vi "Zaber Beginner - Send Commands in a Loop.vi"() -> ()   [LabVIEW 2020]
doc: "You can repeat commands using for loop or while loop structures. This example shows how to use a for loop to replace the five <code>Move Relative -10000</code> commands in the previous example.\nNote that the error line needs to use a shift register in the loop, so that an error will get carried forward through later iterations.\nNow that you've seen two, here are some features common to most of our examples:\n* Place error and COM port wires in a straight line across the bottom. This is the main data flow of the diagram.\n* Start with Initialize to set timeouts and other things, and end with Close. If you don't use Close, Labview won't complain but other applications won't be able to use the COM port."
uses:
  Public/Utility/Request.ctl
  ZaberTSeries.lvlib
panel:
  in  "VISA resource name":refnum<visa-resource-name>
  # "This behaves exactly the same as the previous example,\nbut the block diagram uses a loop.\nType Ctrl-E to see how the block diagram is wired."
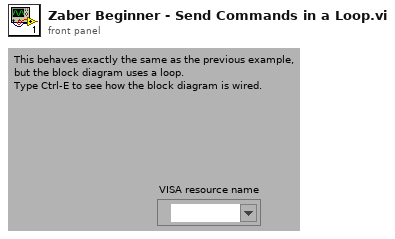
[diagram p1: front panel]
types:
  T1 = typedef "ZaberTSeries.lvlib/Request.ctl" = cluster{"Device Number":u8, "Command":u8, "Data":i32, "Response Count":i32}
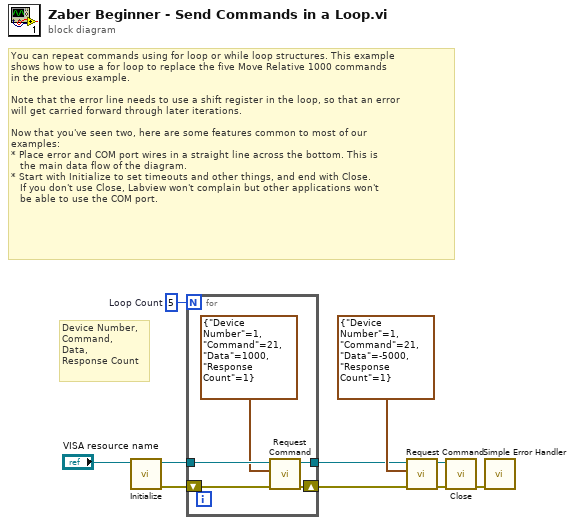
[diagram p0: block diagram]
diagram:
  w1 = 5  # Loop Count
  # "You can repeat commands using for loop or while loop structures. This example\nshows how to use a for loop to replace the five Move Relative 1000 commands \nin the previous example.\n\nNote that the error line needs to use a shift register in the loop, so that an error\nwill get carried forward through later iterations.\n\nNow that you've seen two, here are some features common to most of our\nexamples:\n* Place error and COM port wires in a straight line across the bottom. This is\n   the main data flow of the diagram.\n* Start with Initialize to set timeouts and other things, and end with Close. \n   If you don't use Close, Labview won't complain but other applications won't\n   be able to use the COM port."
  # "Device Number,\nCommand,\nData,\nResponse Count"
  n1 = call "Initialize.vi"("VISA resource name"="VISA resource name") -> ("error out"=w2:errorcluster, "VISA resource name out"=w3:refnum<visa-resource-name>)  [unwired: 8 in, 1 out]
  n2 = for {
    N: w1 -> [_]
    tunnel: w3 -> [w14]
    tunnel: [w12] -> w5
    shift-right: [w11] -> w4
    shift-left: w2 -> [w15]
    n3 = call "Request Command.vi"("error in (no error)"=w15, "Request"=T1 {"Device Number"=1, "Command"=21, "Data"=1000, "Response Count"=1}, "VISA resource name"=w14) -> ("error out"=w11:errorcluster, "VISA resource name out"=w12:refnum<visa-resource-name>)  [unwired: 5 in, 2 out]
  }
  n4 = call "Request Command.vi"("error in (no error)"=w4, "Request"=T1 {"Device Number"=1, "Command"=21, "Data"=-5000, "Response Count"=1}, "VISA resource name"=w5) -> ("error out"=w8:errorcluster, "VISA resource name out"=w9:refnum<visa-resource-name>)  [unwired: 5 in, 2 out]
  n5 = call "Close.vi"("error in (no error)"=w8, "VISA resource name"=w9) -> ("error out"=w10:errorcluster)  [unwired: 8 in, 1 out]
  n6 = call <vilib>:"Simple Error Handler.vi"("error in (no error)"=w10) -> ()  [unwired: 4 in, 5 out]
